vi "Construct Tx Gen.vi"(5 "async loop rate hz":dbl, 7 "error in (no error)":errorcluster, 9 "TX Parameters":T2={"channel #"=0, "channel handle"=0, "InstrumentHandle_board"=0, "InstrumentHandle_port"=0, "channel settings"={"Tx Board"=0, "Tx Port"=0, "Payload Parameter Array"=[], "QueueSizeIn"=1, "Count"=0, "StartMode"=0}, "PayloadMap"={}, "RawFrameMap"={}} {"channel settings"."Payload Parameter Array"."Parameters"."encoding" items=["BNR", "BCD", "Discrete"]}, 10 "custom device ref in":T1=18446744073709551615 format="%.0x") -> (0 "error out":errorcluster, 2 "Tx Execution Unit out":refnum<class "Tx Generic Execution Unit.lvclass">, 3 "custom device ref out":T1=18446744073709551615 format="%.0x")   [LabVIEW 2020, in "AIM ARINC 664 Engine.lvlib" / "Implementation.lvlib" / "Tx Generic Execution Unit.lvclass"]
uses:
  Tx Generic Execution Unit.lvclass
  C:/Users/Administrator/Desktop/GIT/niveristand-aim-arinc664-custom-device/Source/Custom Device Support/Engine/Implementation/Execution Unit/Execution Unit.lvclass
  Shared/hardware_channels_tx.ctl
  Shared/channel_settings_tx.ctl
  Shared/Frame Payload Parameters.ctl
  Shared/Encoding (Arinc664).ctl
  Shared/RawFrame_entry.ctl
  <instrlib>/AIM GmbH/_AIM 664/_controls/queue_header_generic.ctl
  <vilib>/NI VeriStand/Custom Device API/Custom Device Item Ref.ctl
  Tx Generic Execution Unit.lvclass/Tx Generic Execution Unit.ctl
  Execution Unit/Execution Unit.lvclass
  Execution Unit Factory/Execution Unit Factory.lvclass
  <vilib>/NI VeriStand/Custom Device API/Custom Device API.lvlib
  <instrlib>/AIM GmbH/_AIM 664/AIM664LV.lvlib
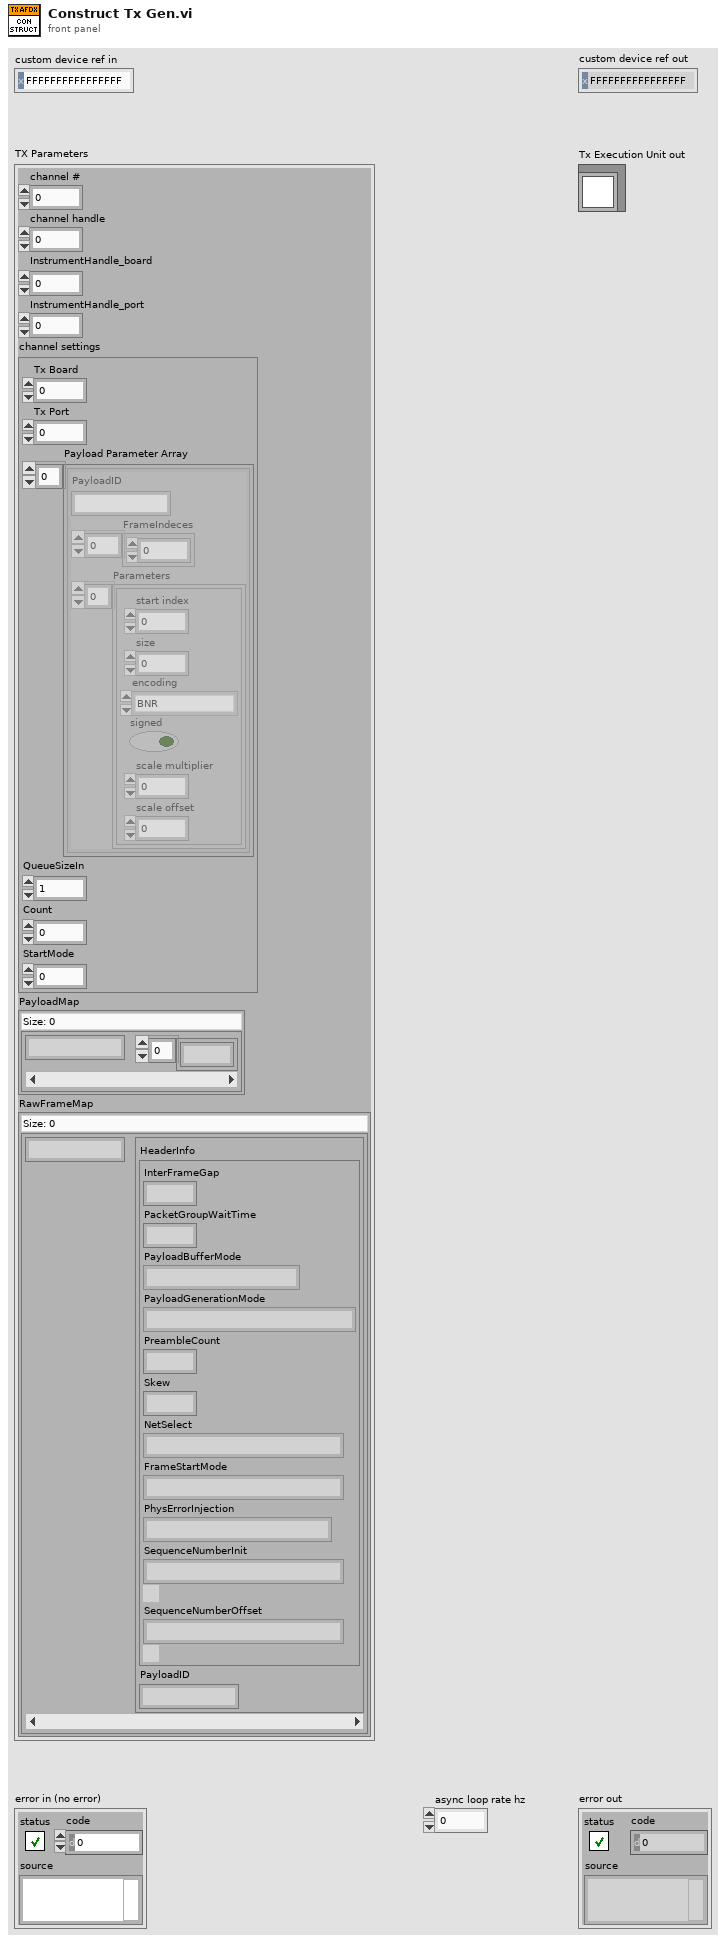
[diagram p1: front panel]
types:
  T1 = typedef "Custom Device API.lvlib/Custom Device Item Ref.ctl" = u64
  T2 = typedef "hardware_channels_tx.ctl" = cluster{"channel #":u16, "channel handle":u64, "InstrumentHandle_board":u32, "InstrumentHandle_port":u32, "channel settings":T3, "PayloadMap":map{string, u8[]}, "RawFrameMap":map{string, T6}}
  T3 = typedef "channel_settings_tx.ctl" = cluster{"Tx Board":u32, "Tx Port":u32, "Payload Parameter Array":T4[], "QueueSizeIn":u32, "Count":u32, "StartMode":u32}
  T4 = typedef "Frame Payload Parameters.ctl" = cluster{"PayloadID":string, "FrameIndeces":u32[], "Parameters":cluster{"start index":i32, "size":i32, "encoding":T5, "signed":bool, "scale multiplier":dbl, "scale offset":dbl}[]}
  T5 = typedef "Encoding (Arinc664).ctl" = u16
  T6 = typedef "RawFrame_entry.ctl" = cluster{"HeaderInfo":T7, "PayloadID":string}
  T7 = typedef "AIM664LV.lvlib/queue_header_generic.ctl" = cluster{"InterFrameGap":u32, "PacketGroupWaitTime":u32, "PayloadBufferMode":u8, "PayloadGenerationMode":u8, "PreambleCount":u8, "Skew":u32, "NetSelect":u8, "FrameStartMode":u8, "PhysErrorInjection":u32, "SequenceNumberInit":u16, "SequenceNumberOffset":u16}
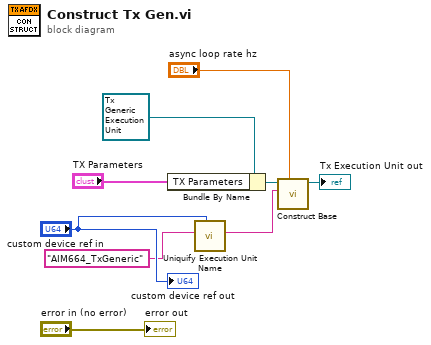
[diagram p0: block diagram]
diagram:
  n1 = Bundle By Name(cluster=refnum<class "Tx Generic Execution Unit.lvclass"> refnum ("Communication Bus Template Interfaces:Implementation.lvlib:Tx Execution Unit.lvclass"), "TX Parameters"="TX Parameters") -> (w6:refnum<class "Tx Generic Execution Unit.lvclass">)
  n2 = call "Uniquify Execution Unit Name.vi"("custom device ref"="custom device ref in", "execution unit name"="AIM664_TxGeneric") -> ("execution unit name out"=w3:string)  [unwired: 9 in]
  n3 = call "Construct Base.vi"("Execution Unit Implementation (default object)"=w6, "identifier"=w3, "async loop rate hz"="async loop rate hz") -> ("Execution Unit Out"=→"Tx Execution Unit out":refnum<class "Tx Generic Execution Unit.lvclass">)  [unwired: 6 in, 1 out]
  "error out" <- "error in (no error)"
  "custom device ref out" <- "custom device ref in"
